vi "ReceiveServerTimestamp.vi"(8 "error in (no error)":errorcluster, 11 "body":variant) -> (0 "error out":errorcluster, 1 "error code":i32, 3 "timestamp":timestamp, 4 "error info":string)   [LabVIEW 2017, in "ServerComm.lvlib"]
doc: "Returns a timestamp from NI InsightCM Server."
uses:
  <vilib>/addons/InsightCM/Devices/Shared/Common/ServerComm/ServerComm.lvlib
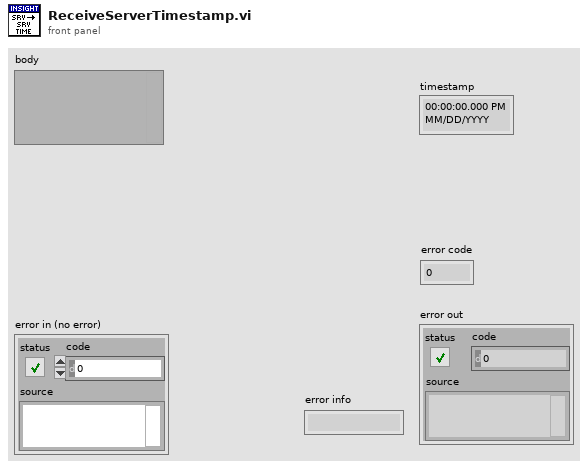
[diagram p1: front panel]
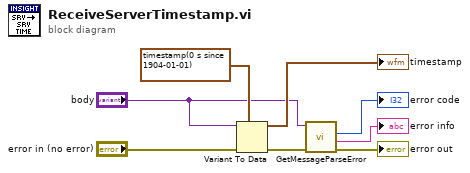
[diagram p0: block diagram]
diagram:
  n1 = Variant To Data(error in="error in (no error)", type=timestamp(0 s since 1904-01-01) ("tcp"), Variant="body") -> (data=→"timestamp":timestamp, error out=w5:errorcluster)
  n2 = call <vilib>:"GetMessageParseError.vi"("error in (no error)"=w5, "body"="body") -> ("error out"=→"error out":errorcluster, "error info"=→"error info":string, "error code"=→"error code":i32)  [unwired: 7 in]
